vi "Auto Intake Loop.vi"(0 "Intake Auto Commands":T1=enum."Idle", 5 "Intake Power":dbl, 7 "Outake Power":dbl) -> (8 "Intake State":T1, 10 "Proposed Power":dbl)   [LabVIEW 2016]
uses:
  Common Code/Intake Auto States.ctl
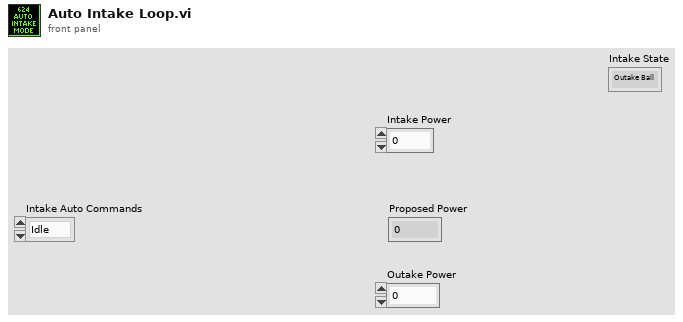
[diagram p1: front panel]
types:
  T1 = typedef "Intake Auto States.ctl" = enum16{"Outake Ball", "Idle", "Load Ball"}
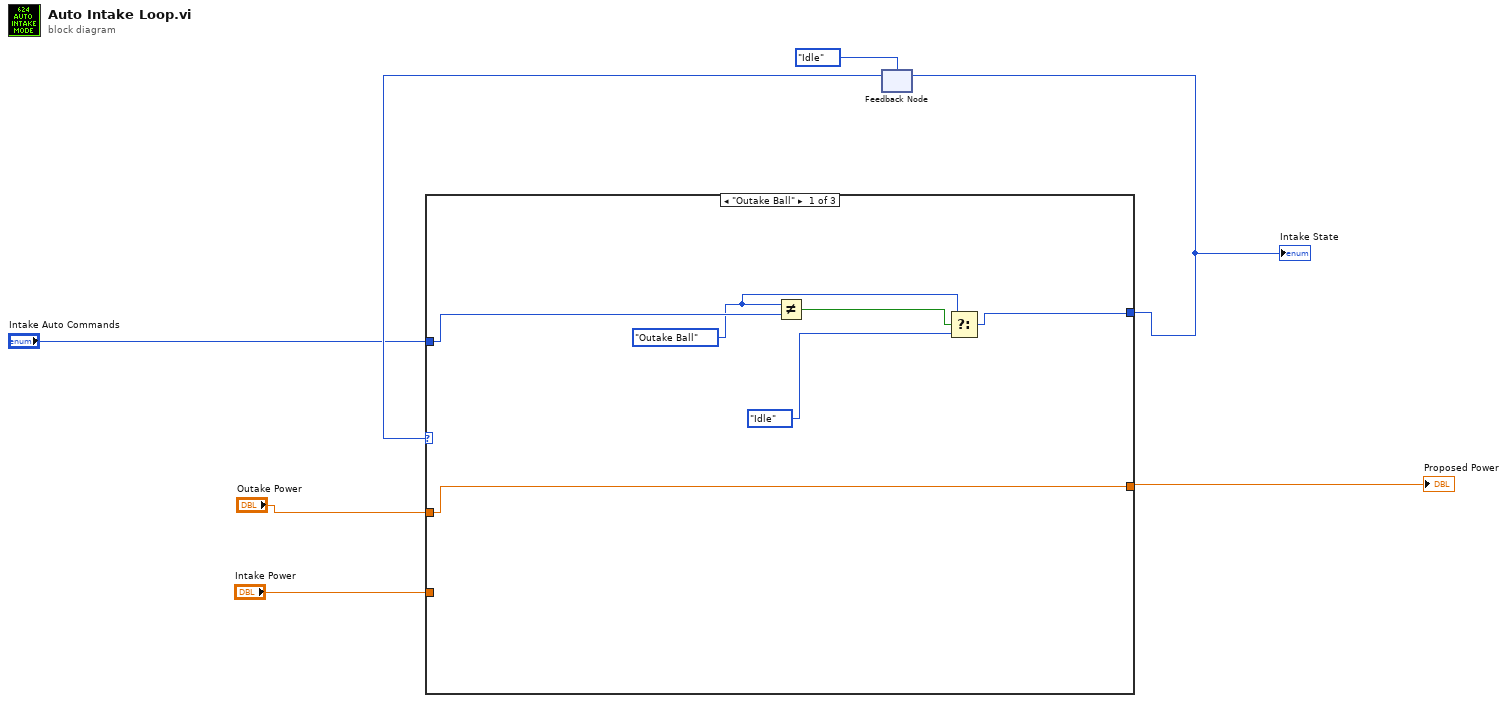
[diagram p0: block diagram]
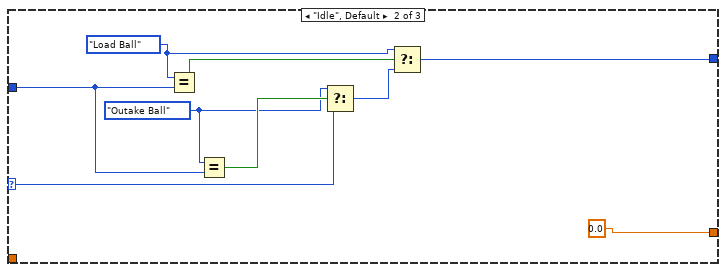
[diagram p2: hidden frame]
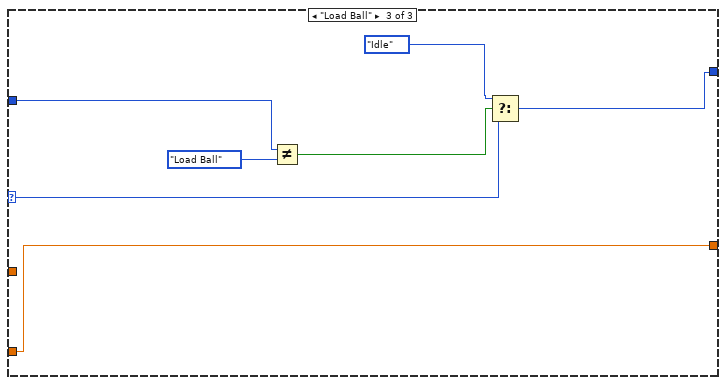
[diagram p3: hidden frame]
diagram:
  n1 = feedback #1(Intake_Auto_States."Idle" ("Intake Auto Commands")) -> (w6:T1)
  n2 = case shown="\"Outake Ball\"" w6 {
    selector: w6 -> [_ w15 w24]
    tunnel: "Intake Auto Commands" -> [w12 w16 w29]
    tunnel: [w8 w20 w25] -> w4
    tunnel: [w9 0.0 w23] -> w3
    tunnel: "Outake Power" -> [w9 _ _]
    tunnel: "Intake Power" -> [_ _ w23]
    frame "Outake Ball" {
      w11 = Intake_Auto_States."Outake Ball" ("Intake Auto Commands")
      n3 = Not Equal?(x=w11, y=w12) -> (x != y?=w13:bool)
      n4 = Select(t=w11, s=w13, f=Intake_Auto_States."Idle" ("Intake Auto Commands")) -> (s? t:f=w8:T1)
    }
    frame "Idle", Default {
      w17 = Intake_Auto_States."Outake Ball" ("Intake Auto Commands")
      w21 = Intake_Auto_States."Load Ball" ("Intake Auto Commands")
      n5 = Equal?(x=w21, y=w16) -> (x = y?=w22:bool)
      n6 = Equal?(x=w17, y=w16) -> (x = y?=w18:bool)
      n7 = Select(t=w17, s=w18, f=w15) -> (s? t:f=w19:T1)
      n8 = Select(t=w21, s=w22, f=w19) -> (s? t:f=w20:T1)
    }
    frame "Load Ball" {
      n9 = Not Equal?(x=w29, y=Intake_Auto_States."Load Ball" ("Intake Auto Commands")) -> (x != y?=w27:bool)
      n10 = Select(t=Intake_Auto_States."Idle" ("Intake Auto Commands"), s=w27, f=w24) -> (s? t:f=w25:T1)
    }
  }
  "Proposed Power" <- w3
  "Intake State" <- w4
  n11 = feedback-in #1(w4) -> ()
